vi "TCP2DDE_main.vi"() -> ()   [LabVIEW 2013]
doc: "Stellt ein Verbindung zum angegebenen Host und Port her und liest die vom Server gesendeten Datums- und Zeitwerte. Zuerst werden 4 Bytes gelesen, um die Länge des Strings zu bestimmen, und dann werden die Daten gelesen. Nach dem Klicken auf Stopp sendet das VI ein Zeichen an das Server-VI, um das Beenden der Verbindung zu signalisieren.\n\n<B>Hinweis:</B> Das VI \"Multiple Connections - Server.vi\" wird benötigt."
uses:
  <vilib>/Utility/error.llb/DialogType.ctl
  <vilib>/Utility/error.llb/whitespace.ctl
  <userlib>/_OpenG.lib/comparison/comparison.llb/String Changed__ogtk.vi
panel:
  out "String":string
  in  "Registerkarte":enum32{"TCP2DDE", "Config"}(tab)
  in  "Sample time":u32=500
  out "Boolesch":bool
  out "data 2":string caption="DDE out"
  out "Azimuth":string caption="°"
  out "Elevation":string caption="°"
  out "Satellite Name":string
  out "Uplink Freq.":string
  out "Downlink Freq.":string
  in  "Man enable 2":bool
  out "Mode":string
  in  "Downlink corr.":i32(knob) scale=-100.0..100.0
  in  "Uplink corr.":i32(knob) scale=-100.0..100.0
  in  "Radio Mode":bool
  out "Current downlink Set.":string caption="Hz"
  out "Current Uplink Set.":string caption="Hz"
  in  "Downlink Freq. Man.":i32=437300000 caption="Hz"
  in  "Uplink Freq. Man.":i32=145855000 caption="Hz"
  out "data":string="\r\n" caption="DDE in"
  in  "stop":bool caption="Stopp"
  in  "Cat Control":bool
  in  "Stop Cat Control":bool
  in  "Type of DN":string
  in  "Type of UP":string
  in  "Port":u16=6341
  in  "Machine":string="localhost" caption="Computer"
  in  "OK-Schaltfläche 6":bool
  in  "Fragmental Window name":string="Hamlib Rotorctld"
  in  "stoppdde":bool=TRUE
  out "Pfad":path
  in  "Save Controls":bool
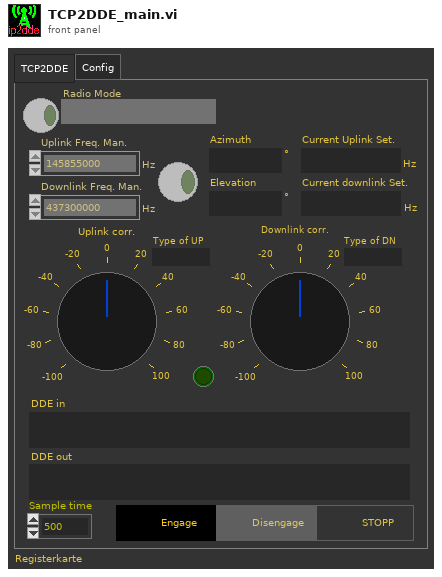
[diagram p1: front panel]
types:
  T1 = enum8{"Enabled", "Disabled", "Disabled and Grayed Out"}
  T2 = typedef "DialogType.ctl" = u16
  T3 = typedef "whitespace.ctl" = u16
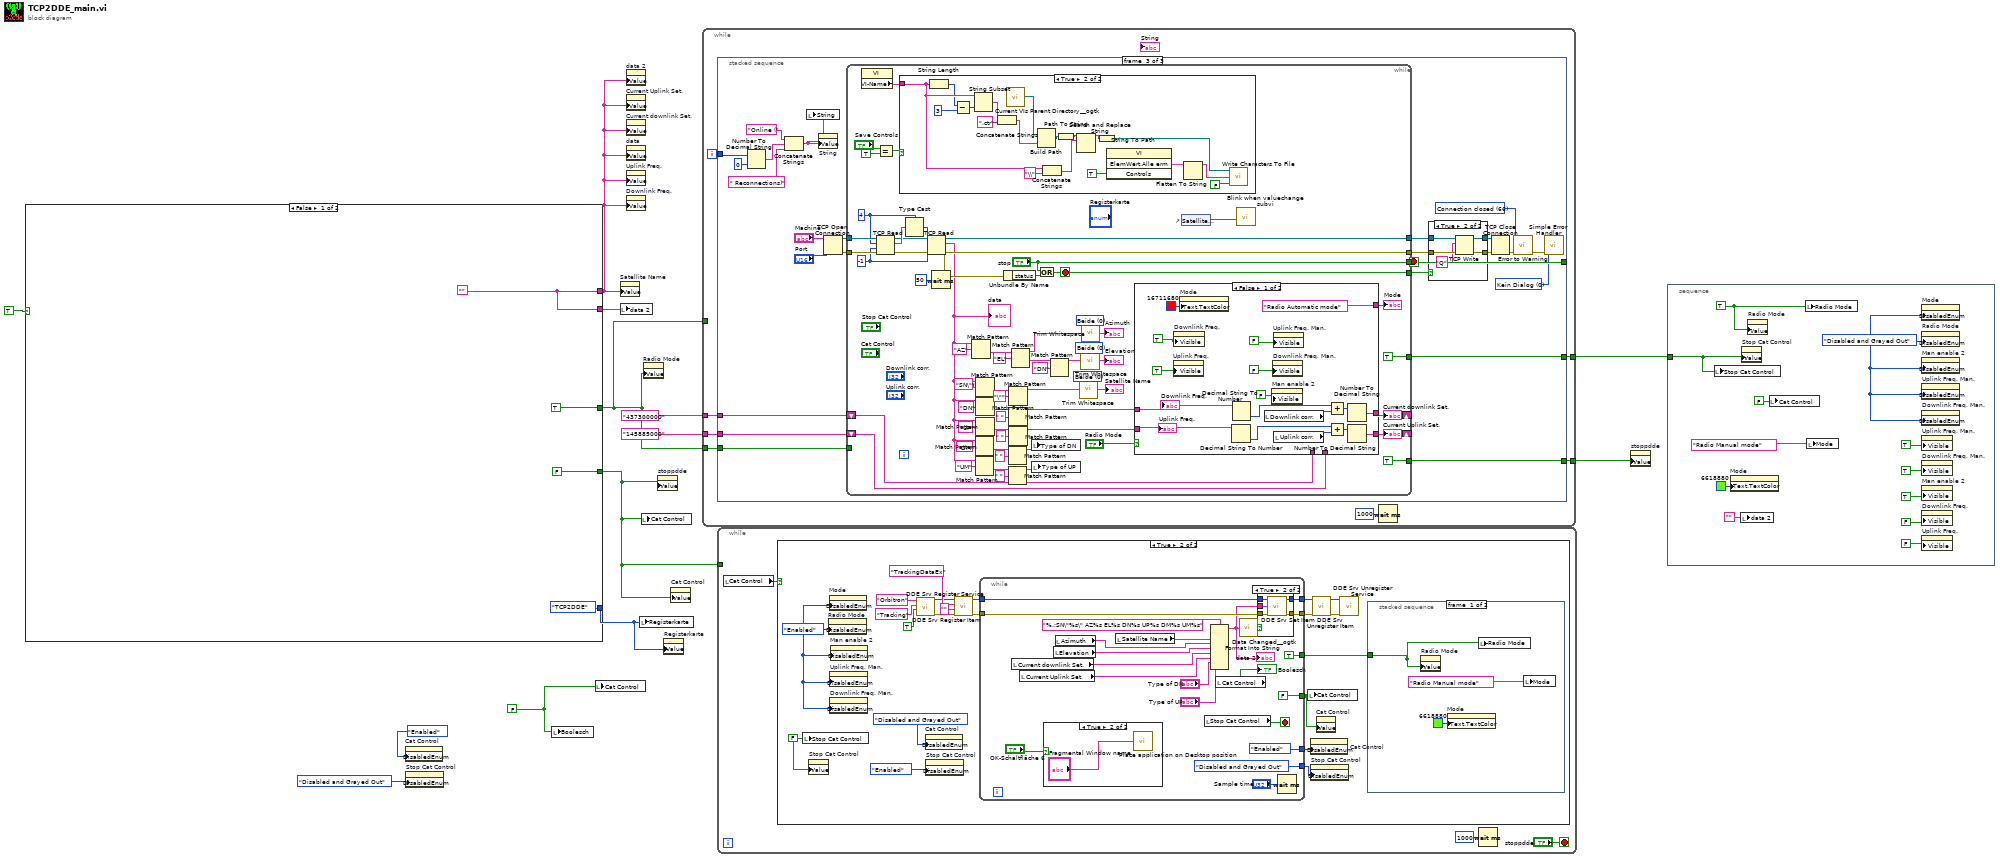
[diagram p0: block diagram]
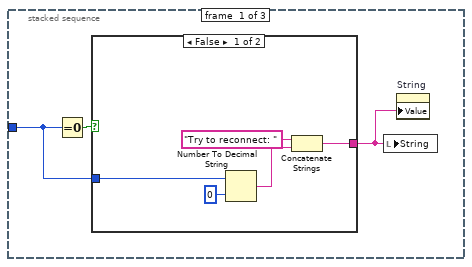
[diagram p2: hidden frame]
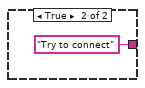
[diagram p3: hidden frame]
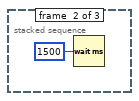
[diagram p4: hidden frame]
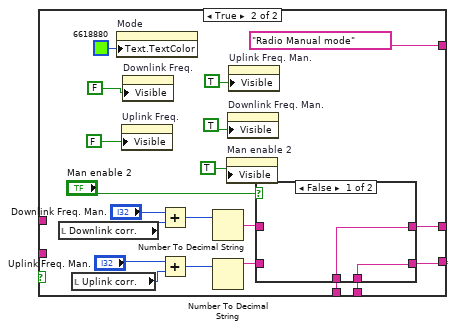
[diagram p6: hidden frame]
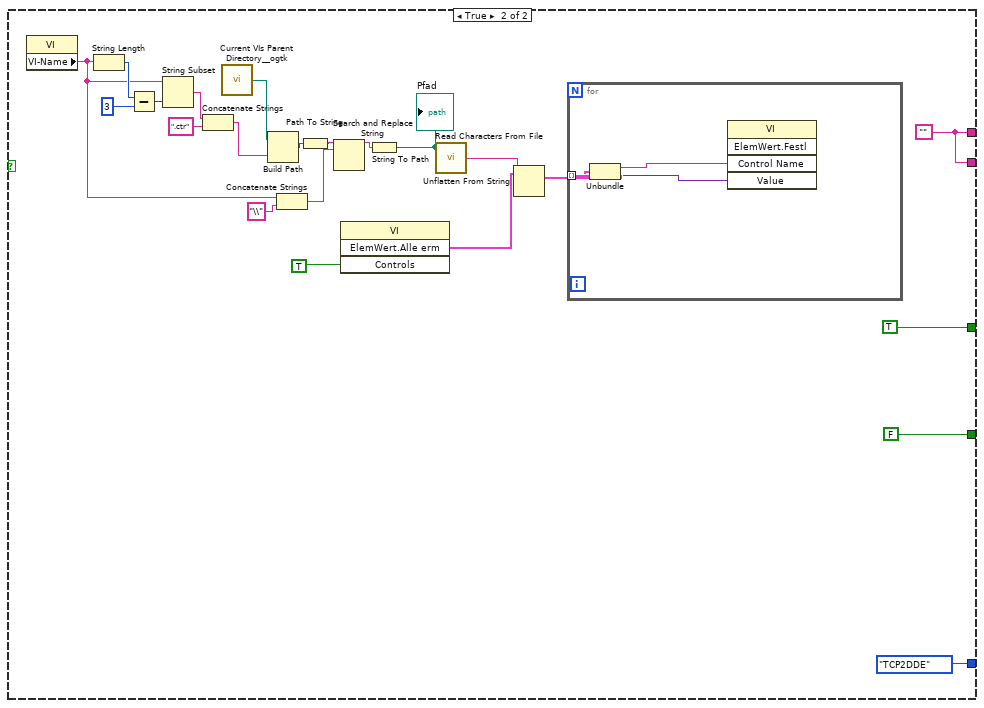
[diagram p9: hidden frame]
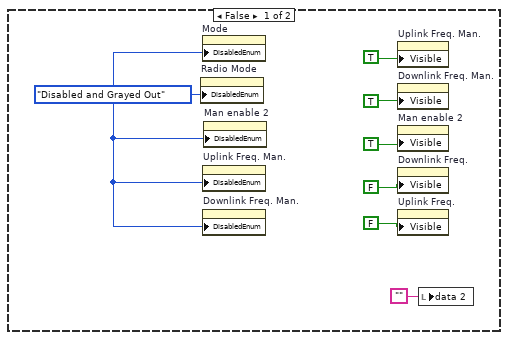
[diagram p10: hidden frame]
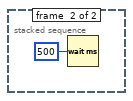
[diagram p11: hidden frame]
diagram:
  w8 = FALSE ("CATCTRL")
  n1 = case shown="False" TRUE {
    tunnel: [TRUE ("Radio Mode") TRUE ("Radio Mode")] -> w1
    tunnel: [FALSE FALSE] -> w2
    tunnel: [w14 w18] -> w9
    tunnel: [enum32{"TCP2DDE", "Config"}."TCP2DDE" ("Registerkarte") enum32{"TCP2DDE", "Config"}."TCP2DDE" ("Registerkarte")] -> w4
    tunnel: [w14 w18] -> w3
    frame False {
      w14 = ""
    }
    frame True {
      w18 = ""
      n2 = property class="VI"() -> ("VI-Name"=w33:string)  [unwired: 2 in, 2 out]
      n3 = String Length(string=w33) -> (length=w34:i32)
      n4 = Subtract(x=w34, y=3) -> (x-y=w36:i32)
      n5 = String Subset(string=w33, length (rest)=w36) -> (substring=w37:string)  [unwired: 1 in]
      n6 = Concatenate Strings(w37, ".ctr" ("String")) -> (w39:string)
      n7 = call "Current VIs Parent Directory__ogtk.vi"() -> ("Parent Directory (+ Relative)"=w22:path)  [unwired: 5 in]
      n8 = Build Path(base path=w22, name or relative path=w39) -> (appended path=w28:path)
      n9 = Concatenate Strings(w33, "\\" ("string")) -> (w32:string)
      n10 = Path To String(path=w28) -> (string=w29:string)
      n11 = Search and Replace String(input string=w29, search string=w32) -> (result string=w30:string)  [unwired: 6 in, 3 out]
      n12 = invoke class="VI" method="ElemWert.Alle erm"("Controls"=TRUE ("controls")) -> ("Get All Control Values Variant"=w27:cluster{"Name":string, "Variant Data":variant}[])  [unwired: 3 in, 3 out]
      n13 = String To Path(string=w30) -> (path=w23:path)
      "Pfad" <- w23
      n14 = call <vilib>:"Read Characters From File.vi"("file path (dialog if empty)"=w23) -> ("character string"=w25:string)  [unwired: 5 in, 3 out]
      n15 = Unflatten From String(type=w27, binary string=w25) -> (value=w26:cluster{"Name":string, "Variant Data":variant}[])  [unwired: 3 in, 2 out]
      n16 = for {
        tunnel: w26 -> [w41] mode=indexing
        n17 = Unbundle(w41) -> ("Name"=w40:string, "Variant Data"=w42:variant)
        n18 = invoke class="VI" method="ElemWert.Festl"("Control Name"=w40, "Value"=w42) -> ()  [unwired: 3 in, 5 out]
      }
    }
  }
  n19 = property on="Cat Control" class="Bool. (strikt)"("DisabledEnum"=T1."Enabled" ("Disabled")) -> ()  [unwired: 2 in, 2 out]
  n20 = property on="Stop Cat Control" class="Bool. (strikt)"("DisabledEnum"=T1."Disabled and Grayed Out" ("Disabled")) -> ()  [unwired: 2 in, 2 out]
  n21 = local write "Boolesch"(w8) -> ()
  n22 = local write "Cat Control"(w8) -> ()
  n23 = property on="Satellite Name" class="Str"("Value"=w9) -> ()  [unwired: 2 in, 2 out]
  n24 = local write "data 2"(w3) -> ()
  n25 = property on="data 2" class="Str"("Value"=w9) -> ()  [unwired: 2 in, 2 out]
  n26 = property on="Current Uplink Set." class="Str"("Value"=w9) -> ()  [unwired: 2 in, 2 out]
  n27 = property on="Current downlink Set." class="Str"("Value"=w9) -> ()  [unwired: 2 in, 2 out]
  n28 = property on="data" class="Str"("Value"=w9) -> ()  [unwired: 2 in, 2 out]
  n29 = property on="Uplink Freq." class="Str"("Value"=w9) -> ()  [unwired: 2 in, 2 out]
  n30 = property on="Downlink Freq." class="Str"("Value"=w9) -> ()  [unwired: 2 in, 2 out]
  n31 = local write "Registerkarte"(w4) -> ()
  n32 = local write "Cat Control"(w2) -> ()
  n33 = property on="Radio Mode" class="Bool. (strikt)"("Value"=w1) -> ()  [unwired: 2 in, 2 out]
  n34 = property on="stoppdde" class="Bool. (strikt)"("Value"=w2) -> ()  [unwired: 2 in, 2 out]
  n35 = property on="Registerkarte" class="RKElem (strikt)"("Value"=w4) -> ()  [unwired: 2 in, 2 out]
  n36 = property on="Cat Control" class="Bool. (strikt)"("Value"=w2) -> ()  [unwired: 2 in, 2 out]
  n37 = while {
    tunnel: [w50] -> w13
    tunnel: "437300000" -> [w49]
    tunnel: "145885000" -> [w48]
    tunnel: w1 -> [w47]
    tunnel: [w46] -> w5
    tunnel: w1 -> [_]
    i -> [w44]
    stop <- w45 stop-if-true
    n38 = stacked-sequence {
      tunnel: [_ _ w74] -> w50
      tunnel: w49 -> [_ _ w73]
      tunnel: w48 -> [_ _ w72]
      tunnel: w47 -> [_ _ w71]
      tunnel: [_ _ w70] -> w46
      tunnel: [_ _ w69] -> w45
      tunnel: w44 -> [w52 _ w63]
      frame #0 {
        n39 = Equal To 0?(x=w52) -> (x = 0?=w53:bool)
        n40 = case shown="False" w53 {
          tunnel: w52 -> [w58 _]
          tunnel: [w54 "Try to connect"] -> w51
          frame False {
            n41 = Number To Decimal String(number=w58, width (-)=i16 0 ("Breite (-)")) -> (decimal integer string=w56:string)
            n42 = Concatenate Strings("Try to reconnect: " ("String"), w56) -> (w54:string)
          }
          frame True {
          }
        }
        n43 = local write "String"(w51) -> ()
        n44 = property on="String" class="Str"("Value"=w51) -> ()  [unwired: 2 in, 2 out]
      }
      frame #1 {
        n45 = Wait (ms)(milliseconds to wait=u32 1500 ("Zu wartende ms")) -> ()  [unwired: 1 out]
      }
      frame #2 {
        w67 = T2 0 items=["Kein Dialog", "OK-Meldung", "Dialog zum Fortsetzen oder Anhalten", "OK-Meldung + Warnungen", "Weiter/Stopp + Warnung"] ("type of dialog (OK msg:1)")
        w75 = 66 items=["No Error", "Argument Error", "Memory Full", "Out of Zone", "End of File", "File Already Open", "Generic File IO Error", "File Not Found", "File Permission Error", "Disk Full", "Duplicate Path", "Too Many Files Open", "Not Enabled", "Resource File Not Found", "Cannot Add Resource", "Resource Not Found", "Image Not Found", "Image Memory Error", "Pen Does Not Exist", "Config Bad Type", "Config Token Not Found", "Config Parse Error", "Config Memory Error", "Bad External Code Format", "Bad External Code Offset", "External Code Not Present", "Null Window", "Destroy Window Mixup", "Null Menu", "Print Aborted", "Bad Print Record", "Print Driver Error", "Windows Error During Print", "Memory Error During Print", "Print Dialog Error", "Generic Print Error", "Invalid Device Refnum", "Device Not Found", "Device Parameter Error", "Device Unit Error", "Can't Open Device", "Device Call Aborted", "Generic Error", "Cancelled By User", "Object ID Too Low", "Object ID Too High", "Object Not In Heap", "Unknown Heap", "Bad DefProc ID", "DefProc Not In Table", "Message Out Of Range", "Null Method", "Unknown Message", "Manager Call Not Supported", "Bad address", "Connection In progress", "Connection timed out", "Connection is already in progress", "Network attribute not supported", "Network error", "Address in use", "System out of memory", "Connection aborted", "Connection refused", "Connection is not connected", "Connection is already connected", "Connection closed", "Initialize error (interapplication manager)", "Bad occurrence", "Wait on unbound occurrence handler", "Occurrence queue overflow", "Bad path", "Semaphore not signaled", "Unrecognized type (interapplication manager)"] ("1st Error to Convert")
        n46 = Number To Decimal String(number=w63, width (-)=i16 0 ("Breite (-)")) -> (decimal integer string=w65:string)
        n47 = Concatenate Strings("Online (" ("String"), w65, " Reconnections)" ("String")) -> (w61:string)
        n48 = local write "String"(w61) -> ()
        n49 = property on="String" class="Str"("Value"=w61) -> ()  [unwired: 2 in, 2 out]
        n50 = TCP Open Connection(address="Machine", remote port or service name="Port") -> (connection ID=w83:refnum<k5>, error out=w82:errorcluster)  [unwired: 1 in, 2 out]
        n51 = while {
          tunnel: ["stop"] -> w69
          tunnel: [w139] -> w81
          tunnel: [w137] -> w79
          tunnel: w82 -> [w145]
          tunnel: w83 -> [w146]
          tunnel: [TRUE] -> w74
          shift-right: [w97] -> _
          shift-left: w73 -> [w94]
          shift-right: [w96] -> _
          shift-left: w72 -> [w95]
          tunnel: w71 -> [_]
          tunnel: [TRUE] -> w70
          tunnel: [w87] -> w68
          stop <- w87 stop-if-true
          w100 = T3 0 items=["Beide", "String-Anfang", "String-Ende"] ("location (both)")
          w103 = T3 0 items=["Beide", "String-Anfang", "String-Ende"] ("location (both)")
          w104 = T3 0 items=["Beide", "String-Anfang", "String-Ende"] ("location (both)")
          w138 = -1
          w144 = 4
          n52 = property class="VI"() -> ("VI-Name"=w93:string)  [unwired: 2 in, 2 out]
          n53 = TCP Read(connection ID=w146, bytes to read=w144, error in (no error)=w145, 9:w138) -> (connection ID out=w140:refnum<k5>, data out=w143:string, error out=w142:errorcluster)  [unwired: 1 out]
          n54 = Equal?(x="Save Controls", y=TRUE) -> (x = y?=w92:bool)
          n55 = case shown="True" w92 {
            tunnel: w93 -> [_ w164]
            frame False {
            }
            frame True {
              n56 = String Length(string=w164) -> (length=w158:i32)
              n57 = Subtract(x=w158, y=3) -> (x-y=w160:i32)
              n58 = String Subset(string=w164, length (rest)=w160) -> (substring=w161:string)  [unwired: 1 in]
              n59 = Concatenate Strings(w161, ".ctr" ("String")) -> (w163:string)
              n60 = call "Current VIs Parent Directory__ogtk.vi"() -> ("Parent Directory (+ Relative)"=w148:path)  [unwired: 5 in]
              n61 = Build Path(base path=w148, name or relative path=w163) -> (appended path=w153:path)
              n62 = Concatenate Strings(w164, "\\" ("string")) -> (w157:string)
              n63 = Path To String(path=w153) -> (string=w154:string)
              n64 = Search and Replace String(input string=w154, search string=w157) -> (result string=w155:string)  [unwired: 6 in, 3 out]
              n65 = String To Path(string=w155) -> (path=w147:path)
              n66 = invoke class="VI" method="ElemWert.Alle erm"("Controls"=TRUE ("controls")) -> ("Get All Control Values Variant"=w151:cluster{"Name":string, "Variant Data":variant}[])  [unwired: 3 in, 3 out]
              n67 = Flatten To String(anything=w151) -> (data string=w150:string)  [unwired: 3 in, 2 out]
              n68 = call <vilib>:"Write Characters To File.vi"("append to file? (new file:F)"=FALSE, "character string"=w150, "file path (dialog if empty)"=w147) -> ()  [unwired: 2 in, 1 out]
            }
          }
          n69 = Type Cast(type=w144, x=w143) -> (*(type *) &x=w141:i32)
          n70 = TCP Read(connection ID=w140, bytes to read=w141, error in (no error)=w142, 9:w138) -> (connection ID out=w139:refnum<k5>, data out=w111:string, error out=w137:errorcluster)  [unwired: 1 out]
          "data" <- w111
          n71 = Wait (ms)(milliseconds to wait=u32 50 ("Zu wartende ms")) -> ()  [unwired: 1 out]
          n72 = Match Pattern(string=w111, regular expression="AZ" ("Regulärer Ausdruck")) -> (after substring=w133:string)  [unwired: 1 in, 3 out]
          n73 = Match Pattern(string=w111, regular expression="DM" ("Regulärer Ausdruck")) -> (after substring=w110:string)  [unwired: 1 in, 3 out]
          n74 = Match Pattern(string=w111, regular expression="UM" ("Regulärer Ausdruck")) -> (after substring=w114:string)  [unwired: 1 in, 3 out]
          n75 = Match Pattern(string=w111, regular expression="SN\"" ("Regulärer Ausdruck")) -> (after substring=w122:string)  [unwired: 1 in, 3 out]
          n76 = Match Pattern(string=w111, regular expression="DN" ("Regulärer Ausdruck")) -> (after substring=w125:string)  [unwired: 1 in, 3 out]
          n77 = Match Pattern(string=w111, regular expression="UP" ("Regulärer Ausdruck")) -> (after substring=w128:string)  [unwired: 1 in, 3 out]
          n78 = Unbundle By Name(w137) -> ("status"=w136:bool)
          n79 = Match Pattern(string=w110, regular expression=" " ("Regulärer Ausdruck")) -> (before substring=w108:string)  [unwired: 1 in, 3 out]
          n80 = Match Pattern(string=w114, regular expression=" " ("Regulärer Ausdruck")) -> (before substring=w109:string)  [unwired: 1 in, 3 out]
          n81 = Match Pattern(string=w122, regular expression="\"" ("Regulärer Ausdruck")) -> (before substring=w99:string)  [unwired: 1 in, 3 out]
          n82 = Match Pattern(string=w125, regular expression=" " ("Regulärer Ausdruck")) -> (before substring=w119:string)  [unwired: 1 in, 3 out]
          n83 = Match Pattern(string=w128, regular expression=" " ("Regulärer Ausdruck")) -> (before substring=w118:string)  [unwired: 1 in, 3 out]
          n84 = Match Pattern(string=w133, regular expression="EL" ("Regulärer Ausdruck")) -> (before substring=w102:string, after substring=w131:string)  [unwired: 1 in, 2 out]
          n85 = local write "Type of DN"(w108) -> ()
          n86 = local write "Type of UP"(w109) -> ()
          n87 = Or(x="stop", y=w136) -> (x .or. y?=w87:bool)
          n88 = Match Pattern(string=w131, regular expression="DN" ("Regulärer Ausdruck")) -> (before substring=w106:string)  [unwired: 1 in, 3 out]
          n89 = call <vilib>:"Trim Whitespace.vi"("string"=w99, "location (both)"=w100) -> ("trimmed string"=→"Satellite Name":string)
          n90 = call <vilib>:"Trim Whitespace.vi"("string"=w106, "location (both)"=w104) -> ("trimmed string"=→"Elevation":string)
          n91 = call <vilib>:"Trim Whitespace.vi"("string"=w102, "location (both)"=w103) -> ("trimmed string"=→"Azimuth":string)
          n92 = case shown="False" "Radio Mode" {
            tunnel: w118 -> [w166 _]
            tunnel: w119 -> [w167 _]
            tunnel: [w171 w197] -> w97
            tunnel: [w170 w196] -> w96
            tunnel: ["Radio Automatic mode" "Radio Manual mode"] -> w120
            tunnel: w95 -> [_ w184]
            tunnel: w94 -> [_ w183]
            frame False {
              n93 = property on="Uplink Freq." class="Str"("Visible"=TRUE) -> ()  [unwired: 2 in, 2 out]
              n94 = property on="Downlink Freq." class="Str"("Visible"=TRUE) -> ()  [unwired: 2 in, 2 out]
              n95 = property on="Mode" class="Str"("Text.TextColor"=u32 16711680) -> ()  [unwired: 2 in, 2 out]
              n96 = Decimal String To Number(string=w166) -> (number=w177:i32)  [unwired: 2 in, 1 out]
              n97 = Decimal String To Number(string=w167) -> (number=w176:i32)  [unwired: 2 in, 1 out]
              n98 = local read "Downlink corr."() -> (w172:i32)
              n99 = property on="Man enable 2" class="Bool."("Visible"=FALSE ("Sichtbar")) -> ()  [unwired: 2 in, 2 out]
              n100 = property on="Downlink Freq. Man." class="DigWert (strikt)"("Visible"=FALSE) -> ()  [unwired: 2 in, 2 out]
              n101 = property on="Uplink Freq. Man." class="DigWert (strikt)"("Visible"=FALSE) -> ()  [unwired: 2 in, 2 out]
              n102 = local read "Uplink corr."() -> (w173:i32)
              n103 = Add(x=w176, y=w172) -> (x+y=w175:i32)
              n104 = Add(x=w177, y=w173) -> (x+y=w174:i32)
              n105 = Number To Decimal String(number=w175) -> (decimal integer string=w171:string)  [unwired: 1 in]
              n106 = Number To Decimal String(number=w174) -> (decimal integer string=w170:string)  [unwired: 1 in]
              "Downlink Freq." <- w167
              "Uplink Freq." <- w166
            }
            frame True {
              n107 = local read "Downlink corr."() -> (w193:i32)
              n108 = local read "Uplink corr."() -> (w188:i32)
              n109 = property on="Mode" class="Str"("Text.TextColor"=u32 6618880) -> ()  [unwired: 2 in, 2 out]
              n110 = property on="Uplink Freq." class="Str"("Visible"=FALSE) -> ()  [unwired: 2 in, 2 out]
              n111 = property on="Downlink Freq." class="Str"("Visible"=FALSE) -> ()  [unwired: 2 in, 2 out]
              n112 = Add(x="Downlink Freq. Man.", y=w193) -> (x+y=w192:i32)
              n113 = Add(x="Uplink Freq. Man.", y=w188) -> (x+y=w190:i32)
              n114 = Number To Decimal String(number=w192) -> (decimal integer string=w191:string)  [unwired: 1 in]
              n115 = Number To Decimal String(number=w190) -> (decimal integer string=w187:string)  [unwired: 1 in]
              n116 = property on="Man enable 2" class="Bool."("Visible"=TRUE ("Sichtbar")) -> ()  [unwired: 2 in, 2 out]
              n117 = property on="Downlink Freq. Man." class="DigWert (strikt)"("Visible"=TRUE) -> ()  [unwired: 2 in, 2 out]
              n118 = property on="Uplink Freq. Man." class="DigWert (strikt)"("Visible"=TRUE) -> ()  [unwired: 2 in, 2 out]
              n119 = case shown="False" "Man enable 2" {
                tunnel: [w202 w205] -> w197
                tunnel: w191 -> [_ w205]
                tunnel: w187 -> [_ w204]
                tunnel: [w203 w204] -> w196
                tunnel: w184 -> [w203 _]
                tunnel: w183 -> [w202 _]
                frame False {
                }
                frame True {
                }
              }
            }
          }
          "Mode" <- w120
          "Current downlink Set." <- w97
          "Current Uplink Set." <- w96
          n120 = control-ref of="Satellite Name"() -> (w88:refnum<vi>)
          n121 = call "Blink when valuechange subvi.vi"("Indicator or ctrl to look up value change"=w88) -> ()  [unwired: 9 in, 2 out]
        }
        n122 = case shown="True" w68 {
          tunnel: w81 -> [w207 w212]
          tunnel: [w207 w210] -> w80
          tunnel: w79 -> [w206 w211]
          tunnel: [w206 w209] -> w78
          frame False {
          }
          frame True {
            n123 = TCP Write(connection ID=w212, data in="Q", error in (no error)=w211) -> (connection ID out=w210:refnum<k5>, error out=w209:errorcluster)  [unwired: 2 out]
          }
        }
        n124 = TCP Close Connection(connection ID=w80, error in (no error)=w78) -> (error out=w77:errorcluster)  [unwired: 2 out]
        n125 = call <vilib>:"Error to Warning.vi"("1st Error to Convert"=w75, "error in"=w77) -> ("warning out"=w76:errorcluster)  [unwired: 3 in, 10 out]
        n126 = call <vilib>:"Simple Error Handler.vi"("type of dialog (OK msg:1)"=w67, "error in (no error)"=w76) -> ()  [unwired: 8 out]
      }
    }
    n127 = Wait (ms)(milliseconds to wait=u32 1000 ("Zu wartende ms")) -> ()  [unwired: 1 out]
  }
  n128 = while {
    tunnel: w2 -> [_]
    stop <- "stoppdde" stop-if-true
    n129 = local read "Cat Control"() -> (w214:bool)
    n130 = case shown="True" w214 {
      frame False {
        w222 = T1."Disabled and Grayed Out" ("Deaktiviert")
        n131 = property on="Radio Mode" class="Bool. (strikt)"("DisabledEnum"=w222) -> ()  [unwired: 2 in, 2 out]
        n132 = property on="Mode" class="Str"("DisabledEnum"=w222) -> ()  [unwired: 2 in, 2 out]
        n133 = property on="Uplink Freq. Man." class="DigWert (strikt)"("DisabledEnum"=w222) -> ()  [unwired: 2 in, 2 out]
        n134 = property on="Downlink Freq. Man." class="DigWert (strikt)"("DisabledEnum"=w222) -> ()  [unwired: 2 in, 2 out]
        n135 = property on="Man enable 2" class="Bool."("DisabledEnum"=w222) -> ()  [unwired: 2 in, 2 out]
        n136 = property on="Uplink Freq. Man." class="DigWert (strikt)"("Visible"=TRUE) -> ()  [unwired: 2 in, 2 out]
        n137 = property on="Downlink Freq. Man." class="DigWert (strikt)"("Visible"=TRUE) -> ()  [unwired: 2 in, 2 out]
        n138 = property on="Man enable 2" class="Bool."("Visible"=TRUE ("Sichtbar")) -> ()  [unwired: 2 in, 2 out]
        n139 = property on="Downlink Freq." class="Str"("Visible"=FALSE) -> ()  [unwired: 2 in, 2 out]
        n140 = property on="Uplink Freq." class="Str"("Visible"=FALSE) -> ()  [unwired: 2 in, 2 out]
        n141 = local write "data 2"("") -> ()
      }
      frame True {
        w223 = T1."Enabled" ("Deaktiviert")
        w230 = FALSE ("Stop Cat Control")
        n142 = local write "Stop Cat Control"(w230) -> ()
        n143 = property on="Stop Cat Control" class="Bool. (strikt)"("Value"=w230) -> ()  [unwired: 2 in, 2 out]
        n144 = property on="Radio Mode" class="Bool. (strikt)"("DisabledEnum"=w223) -> ()  [unwired: 2 in, 2 out]
        n145 = property on="Mode" class="Str"("DisabledEnum"=w223) -> ()  [unwired: 2 in, 2 out]
        n146 = property on="Uplink Freq. Man." class="DigWert (strikt)"("DisabledEnum"=w223) -> ()  [unwired: 2 in, 2 out]
        n147 = property on="Downlink Freq. Man." class="DigWert (strikt)"("DisabledEnum"=w223) -> ()  [unwired: 2 in, 2 out]
        n148 = property on="Man enable 2" class="Bool."("DisabledEnum"=w223) -> ()  [unwired: 2 in, 2 out]
        n149 = call <vilib>:"DDE Srv Register Service.vi"("allow dynamic items"=TRUE, "topic"="Tracking", "service"="Orbitron") -> ("error out"=w233:errorcluster, "service refnum"=w234:u32)  [unwired: 5 in]
        n150 = property on="Cat Control" class="Bool. (strikt)"("DisabledEnum"=T1."Disabled and Grayed Out" ("Disabled")) -> ()  [unwired: 2 in, 2 out]
        n151 = property on="Stop Cat Control" class="Bool. (strikt)"("DisabledEnum"=T1."Enabled" ("Disabled")) -> ()  [unwired: 2 in, 2 out]
        n152 = call <vilib>:"DDE Srv Register Item.vi"("error in (no error)"=w233, "value"="", "item"="TrackingDataEx", "service refnum"=w234) -> ("error out"=w236:errorcluster, "item refnum"=w235:u32)  [unwired: 4 in]
        n153 = while {
          tunnel: w235 -> [w269]
          tunnel: w236 -> [w268]
          tunnel: [w267] -> w237
          tunnel: [w266] -> w238
          tunnel: [FALSE] -> w229
          tunnel: [T1."Enabled" ("Disabled")] -> w228
          tunnel: [T1."Disabled and Grayed Out" ("Disabled")] -> w227
          tunnel: [TRUE] -> w224
          stop <- w252 stop-if-true
          n154 = local read "Current downlink Set."() -> (w259:string)
          n155 = local read "Current Uplink Set."() -> (w258:string)
          n156 = case shown="True" "OK-Schaltfläche 6" {
            frame False {
            }
            frame True {
              n157 = call "Place application on Desktop position.vi"("Fragmental Window name"="Fragmental Window name") -> ()  [unwired: 5 in]
            }
          }
          n158 = local read "Elevation"() -> (w260:string)
          n159 = local read "Azimuth"() -> (w261:string)
          n160 = local read "Satellite Name"() -> (w262:string)
          n161 = local read "Stop Cat Control"() -> (w252:bool)
          n162 = Format Into String(format string="%.;SN\"%s\" AZ%s EL%s DN%s UP%s DM%s UM%s", w262, w261, w260, w259, w258, "Type of DN", "Type of UP") -> (resulting string=w255:string)  [unwired: 2 in, 1 out]
          "data 2" <- w255
          n163 = local read "Cat Control"() -> (→"Boolesch":bool)
          n164 = call-poly <userlib>:"Data Changed__ogtk.vi"("String"=w255) -> ("Changed"=w264:bool)
          n165 = case shown="True" w264 {
            tunnel: w269 -> [w272 w277]
            tunnel: w268 -> [w271 w276]
            tunnel: [w272 w275] -> w267
            tunnel: [w271 w274] -> w266
            tunnel: w255 -> [_ w273]
            frame False {
            }
            frame True {
              n166 = call <vilib>:"DDE Srv Set Item.vi"("error in (no error)"=w276, "value"=w273, "item refnum in"=w277) -> ("error out"=w274:errorcluster, "item refnum out"=w275:u32)  [unwired: 5 in]
            }
          }
          n167 = Wait (ms)(milliseconds to wait="Sample time") -> ()  [unwired: 1 out]
        }
        n168 = local write "Cat Control"(w229) -> ()
        n169 = property on="Cat Control" class="Bool. (strikt)"("DisabledEnum"=w228) -> ()  [unwired: 2 in, 2 out]
        n170 = property on="Stop Cat Control" class="Bool. (strikt)"("DisabledEnum"=w227) -> ()  [unwired: 2 in, 2 out]
        n171 = call <vilib>:"DDE Srv Unregister Item.vi"("error in (no error)"=w238, "item refnum"=w237) -> ("error out"=w240:errorcluster, "service refnum"=w239:u32)  [unwired: 6 in]
        n172 = property on="Cat Control" class="Bool. (strikt)"("Value"=w229) -> ()  [unwired: 2 in, 2 out]
        n173 = call <vilib>:"DDE Srv Unregister Service.vi"("error in (no error)"=w240, "service refnum"=w239) -> ()  [unwired: 7 in, 1 out]
        n174 = stacked-sequence {
          tunnel: w224 -> [w246 _]
          frame #0 {
            n175 = property on="Radio Mode" class="Bool. (strikt)"("Value"=w246) -> ()  [unwired: 2 in, 2 out]
            n176 = property on="Mode" class="Str"("Text.TextColor"=u32 6618880) -> ()  [unwired: 2 in, 2 out]
            n177 = local write "Radio Mode"(w246) -> ()
            n178 = local write "Mode"("Radio Manual mode") -> ()
          }
          frame #1 {
            n179 = Wait (ms)(milliseconds to wait=u32 500 ("Zu wartende ms")) -> ()  [unwired: 1 out]
          }
        }
      }
    }
    n180 = Wait (ms)(milliseconds to wait=u32 1000 ("Zu wartende ms")) -> ()  [unwired: 1 out]
  }
  n181 = property on="stoppdde" class="Bool. (strikt)"("Value"=w13) -> ()  [unwired: 2 in, 2 out]
  n182 = stacked-sequence {
    tunnel: w5 -> [w288]
    frame #0 {
      w284 = T1."Disabled and Grayed Out" ("Deaktiviert")
      w287 = TRUE
      n183 = local write "Stop Cat Control"(w288) -> ()
      n184 = property on="Mode" class="Str"("Text.TextColor"=u32 6618880) -> ()  [unwired: 2 in, 2 out]
      n185 = local write "data 2"("") -> ()
      n186 = property on="Stop Cat Control" class="Bool. (strikt)"("Value"=w288) -> ()  [unwired: 2 in, 2 out]
      n187 = property on="Radio Mode" class="Bool. (strikt)"("Value"=w287) -> ()  [unwired: 2 in, 2 out]
      n188 = local write "Cat Control"(FALSE ("Cat Control")) -> ()
      n189 = local write "Radio Mode"(w287) -> ()
      n190 = local write "Mode"("Radio Manual mode") -> ()
      n191 = property on="Mode" class="Str"("DisabledEnum"=w284) -> ()  [unwired: 2 in, 2 out]
      n192 = property on="Radio Mode" class="Bool. (strikt)"("DisabledEnum"=w284) -> ()  [unwired: 2 in, 2 out]
      n193 = property on="Man enable 2" class="Bool."("DisabledEnum"=w284) -> ()  [unwired: 2 in, 2 out]
      n194 = property on="Uplink Freq. Man." class="DigWert (strikt)"("DisabledEnum"=w284) -> ()  [unwired: 2 in, 2 out]
      n195 = property on="Downlink Freq. Man." class="DigWert (strikt)"("DisabledEnum"=w284) -> ()  [unwired: 2 in, 2 out]
      n196 = property on="Uplink Freq. Man." class="DigWert (strikt)"("Visible"=TRUE) -> ()  [unwired: 2 in, 2 out]
      n197 = property on="Downlink Freq. Man." class="DigWert (strikt)"("Visible"=TRUE) -> ()  [unwired: 2 in, 2 out]
      n198 = property on="Man enable 2" class="Bool."("Visible"=TRUE ("Sichtbar")) -> ()  [unwired: 2 in, 2 out]
      n199 = property on="Downlink Freq." class="Str"("Visible"=FALSE) -> ()  [unwired: 2 in, 2 out]
      n200 = property on="Uplink Freq." class="Str"("Visible"=FALSE) -> ()  [unwired: 2 in, 2 out]
    }
  }
